vi "FrequencyFilter.vi"(0 "Image In":T2, 1 "Color Mode (Color Threshold 1)":u16(ring) items=["RGB", "HSL", "HSV", "HSI"], 2 "Red or Hue Range (Color Threshold 1)":cluster{"Lower value":i32, "Upper value":i32}={"Lower value"=0, "Upper value"=243}, 3 "Green or Sat Range (Color Threshold 1)":cluster{"Lower value":i32, "Upper value":i32}={"Lower value"=229, "Upper value"=255}, 4 "Blue or Luma or Val or Inten Range (Color Threshold 1)":cluster{"Lower value":i32, "Upper value":i32}={"Lower value"=219, "Upper value"=255}, 5 "Low pass/High pass (Low pass) (FFT Filter 2)":bool=TRUE, 6 "Truncation Frequency % (FFT Filter 2)":sgl=5.0, 7 "error in":errorcluster, 8 "Low pass/High pass (Low pass) (FFT Filter 1)":bool, 9 "Truncation Frequency % (FFT Filter 1)":sgl=5.0, 10 "Number of Erosion (Advanced Morphology 2)":i32=5, 11 "Square/Hexa (Square) (Advanced Morphology 2)":bool, 12 "Low Pass/High Pass (Low) (Advanced Morphology 2)":bool) -> (20 "Image Out":T2, 21 "Number of Particles (Particle Analysis 1)":i32, 24 "Centroid":cluster{"X Centroid":sgl, "Y Centroid":sgl} {"Y Centroid" format="%.2f"; "X Centroid" format="%.2f"}, 25 "Calibrated Centroid":cluster{"X":sgl, "Y":sgl} {"Y" format="%.2f"; "X" format="%.2f"}, 26 "Particle Reports (Pixels)":T1(array[cluster]) {"Orientation" format="%.2f"; "Dimensions"."Height" format="%.2f"; "Dimensions"."Width" format="%.2f"; "Center of Mass"."Y" format="%.2f"; "Center of Mass"."X" format="%.2f"; "Bounding Rect"."Bottom" format="%.2f"; "Bounding Rect"."Right" format="%.2f"; "Bounding Rect"."Top" format="%.2f"; "Bounding Rect"."Left" format="%.2f"; "Number of Holes" format="%.2f"; "Area" format="%.2f"}, 27 "error out":errorcluster)   [LabVIEW 2020]
uses:
  <vilib>/vision/Image Controls.llb/IMAQ Image.ctl
  <vilib>/vision/NI_Vision_Development_Module.lvlib
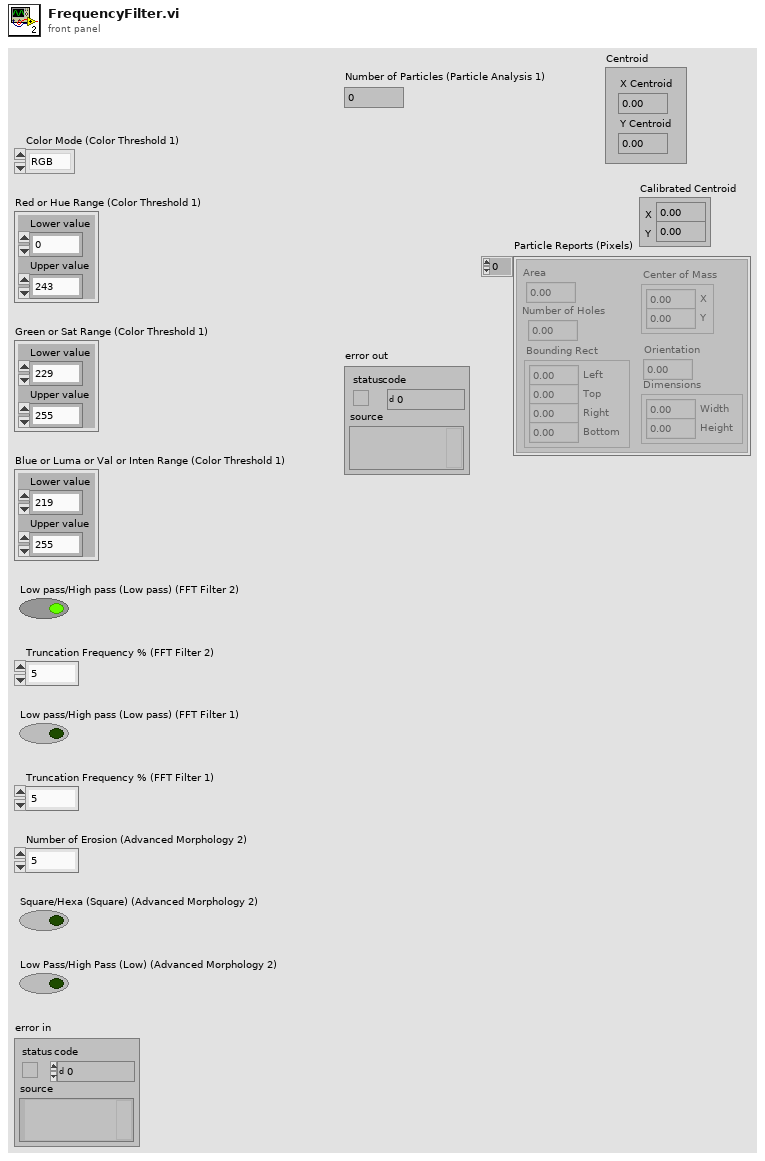
[diagram p1: front panel]
types:
  T1 = cluster{"Area":dbl, "Number of Holes":dbl, "Bounding Rect":cluster{"Left":dbl, "Top":dbl, "Right":dbl, "Bottom":dbl}, "Center of Mass":cluster{"X":dbl, "Y":dbl}, "Orientation":dbl, "Dimensions":cluster{"Width":dbl, "Height":dbl}}[]
  T2 = typedef "IMAQ Image.ctl" = refnum<image>
  T3 = typedef "Image Type" = u32
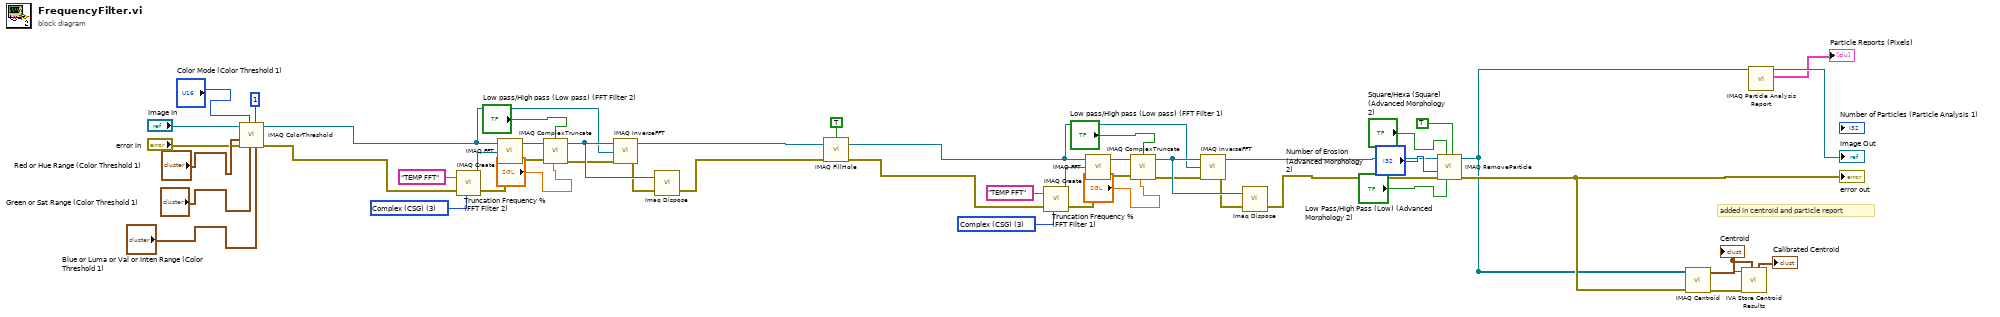
[diagram p0: block diagram]
diagram:
  w13 = T3 3 items=["Grayscale (U8)", "Grayscale (I16)", "Grayscale (SGL)", "Complex (CSG)", "RGB (U32)", "HSL (U32)", "RGB (U64)", "Grayscale (U16)"] ("Image Type")
  w29 = T3 3 items=["Grayscale (U8)", "Grayscale (I16)", "Grayscale (SGL)", "Complex (CSG)", "RGB (U32)", "HSL (U32)", "RGB (U64)", "Grayscale (U16)"] ("Image Type")
  # "added in centroid and particle report"
  n1 = call "IMAQ ColorThreshold"("Blue or Luma or Val or Inten Range"="Blue or Luma or Val or Inten Range (Color Threshold 1)", "Replace Value"=1, "Green or Sat Range"="Green or Sat Range (Color Threshold 1)", "Color Mode"="Color Mode (Color Threshold 1)", "error in (no error)"="error in", "Red or Hue Range"="Red or Hue Range (Color Threshold 1)", "Image Src"="Image In") -> ("error out"=w42:errorcluster, "Image Dst Out"=w32:T2)  [unwired: 1 in, 2 out]
  n2 = call "IMAQ Create"("Image Name"="TEMP FFT", "Image Type"=w29, "error in (no error)"=w42) -> ("New Image"=w40:T2, "error out"=w33:errorcluster)  [unwired: 1 in, 1 out]
  n3 = call "IMAQ FFT"("error in (no error)"=w33, "Image Dst"=w40, "Image Src"=w32) -> ("error out"=w38:errorcluster, "Image Dst Out"=w39:T2)  [unwired: 1 out]
  n4 = call "IMAQ ComplexTruncate"("error in (no error)"=w38, "Truncation Frequency %"="Truncation Frequency % (FFT Filter 2)", "Image Src"=w39, "Low pass/High pass (Low pass)"="Low pass/High pass (Low pass) (FFT Filter 2)") -> ("error out"=w36:errorcluster, "Image Dst Out"=w37:T2)  [unwired: 1 in, 2 out]
  n5 = call "IMAQ InverseFFT"("error in (no error)"=w36, "Image Dst"=w32, "Image Src"=w37) -> ("error out"=w35:errorcluster, "Image Dst Out"=w27:T2)  [unwired: 1 out]
  n6 = call "Imaq Dispose"("Image"=w37, "error in (no error)"=w35) -> ("error out"=w34:errorcluster)  [unwired: 1 in, 3 out]
  n7 = call "IMAQ FillHole"("error in (no error)"=w34, "Image Src"=w27, "Connectivity 4/8 (8)"=TRUE) -> ("error out"=w26:errorcluster, "Image Dst Out"=w16:T2)  [unwired: 1 in, 2 out]
  n8 = call "IMAQ Create"("Image Name"="TEMP FFT", "Image Type"=w13, "error in (no error)"=w26) -> ("New Image"=w24:T2, "error out"=w17:errorcluster)  [unwired: 1 in, 1 out]
  n9 = call "IMAQ FFT"("error in (no error)"=w17, "Image Dst"=w24, "Image Src"=w16) -> ("error out"=w22:errorcluster, "Image Dst Out"=w23:T2)  [unwired: 1 out]
  n10 = call "IMAQ ComplexTruncate"("error in (no error)"=w22, "Truncation Frequency %"="Truncation Frequency % (FFT Filter 1)", "Image Src"=w23, "Low pass/High pass (Low pass)"="Low pass/High pass (Low pass) (FFT Filter 1)") -> ("error out"=w20:errorcluster, "Image Dst Out"=w21:T2)  [unwired: 1 in, 2 out]
  n11 = call "IMAQ InverseFFT"("error in (no error)"=w20, "Image Dst"=w16, "Image Src"=w21) -> ("error out"=w19:errorcluster, "Image Dst Out"=w8:T2)  [unwired: 1 out]
  n12 = call "Imaq Dispose"("Image"=w21, "error in (no error)"=w19) -> ("error out"=w18:errorcluster)  [unwired: 1 in, 3 out]
  n13 = call "IMAQ RemoveParticle"("Connectivity 4/8 (8)"=TRUE, "Low Pass/High Pass (Low)"="Low Pass/High Pass (Low) (Advanced Morphology 2)", "Square/Hexa (Square)"="Square/Hexa (Square) (Advanced Morphology 2)", "error in (no error)"=w18, "Number of Erosion"="Number of Erosion (Advanced Morphology 2)", "Image Src"=w8) -> ("error out"=w4:errorcluster, "Image Dst Out"=w3:T2)  [unwired: 1 in, 3 out]
  "error out" <- w4
  n14 = call "IMAQ Centroid"("error in (no error)"=w4, "Image"=w3) -> ("error out"=w7:errorcluster, "Centroid"=w5:cluster{"X Centroid":sgl, "Y Centroid":sgl})  [unwired: 1 in, 1 out]
  "Centroid" <- w5
  n15 = call <vilib>:"IVA Store Centroid Results.vi"("Centroid in"=w5, "error in (no error)"=w7, "Image in"=w3) -> ("Calibrated Centroid"=→"Calibrated Centroid":cluster{"X":sgl, "Y":sgl})  [unwired: 1 in, 7 out]
  n16 = call "IMAQ Particle Analysis Report"("Image"=w3) -> ("Particle Reports (Pixels)"=→"Particle Reports (Pixels)":T1, "Image Out (duplicate)"=→"Image Out":T2)  [unwired: 5 in, 4 out]
